vi "HAL camera cooler off.vi"() -> (0 "Error?":bool)   [LabVIEW 2015]
uses:
  ATMCD32D.DLL
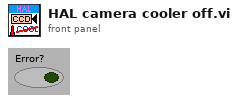
[diagram p1: front panel]
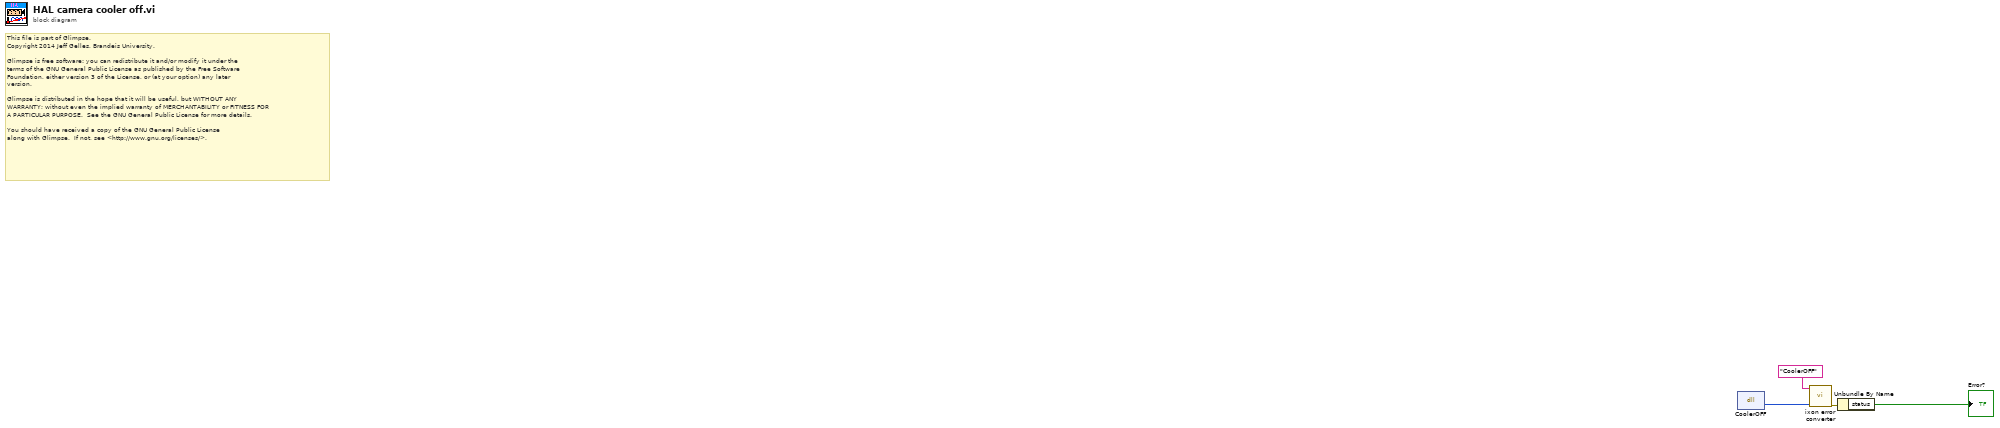
[diagram p0: block diagram]
diagram:
  # "This file is part of Glimpse. \nCopyright 2014 Jeff Gelles, Brandeis University.    \n\nGlimpse is free software: you can redistribute it and/or modify it under the \nterms of the GNU General Public License as published by the Free Software \nFoundation, either version 3 of the License, or (at your option) any later \nversion.\n\nGlimpse is distributed in the hope that it will be useful, but WITHOUT ANY \nWARRANTY; without even the implied warranty of MERCHANTABILITY or FITNESS FOR \nA PARTICULAR PURPOSE.  See the GNU General Public License for more details.\n\nYou should have received a copy of the GNU General Public License\nalong with Glimpse.  If not, see <http://www.gnu.org/licenses/>."
  n1 = dll-call lib="ATMCD32D.DLL" fn="CoolerOFF" label="CoolerOff"() -> (w2:u32)  [unwired: 3 in, 2 out]
  n2 = call "ixon error converter.vi"("Andor error code"=w2, "source"="CoolerOFF") -> ("error out"=w3:errorcluster)  [unwired: 5 out]
  n3 = Unbundle By Name(w3) -> ("status"=→"Error?":bool)
